vi "GetDevice.vi"(10 "EMG Input Device\nProduct Type":string) -> (2 "DAQmx Device Name":tag)   [LabVIEW 2016]
uses:
  <resource>/objmgr/daqmx.rc
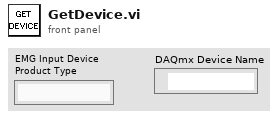
[diagram p1: front panel]
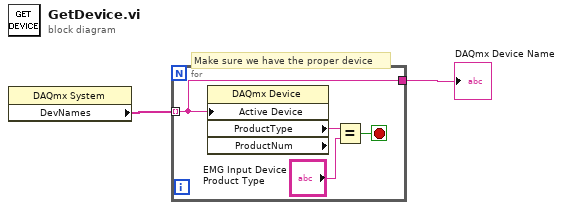
[diagram p0: block diagram]
diagram:
  # "Make sure we have the proper device"
  n1 = property class="DAQmx System"() -> ("DevNames"=w2:tag[])  [unwired: 2 in, 2 out]
  n2 = for {
    tunnel: w2 -> [w3] mode=indexing
    tunnel: [w3] -> w1
    stop <- w4 stop-if-true
    n3 = property class="DAQmx Device" props=["Active Device", "ProductType", "ProductNum"]("Active Device"=w3) -> ("ProductType"=w6:string)  [unwired: 2 in, 3 out]
    n4 = Equal?(x=w6, y="EMG Input Device\nProduct Type") -> (x = y?=w4:bool)
  }
  "DAQmx Device Name" <- w1
